vi "testFailIfEqual.vi"(8 "error in (no error)":errorcluster, 11 "MyFirstTest.lvclass in":refnum<class "MyFirstTest.lvclass">) -> (0 "error out":errorcluster, 3 "MyFirstTest.lvclass out":refnum<class "MyFirstTest.lvclass">)   [LabVIEW 2013, in "MyFirstTest.lvclass"]
doc: "This VI is a demo test -- it ensures that \"dog\" != \"cat\""
uses:
  MyFirstTest.lvclass
panel:
  # "Copyright © 2007 James Kring, Inc. All rights reserved.\n\nAuthor: Jim Kring [jim.kring@jameskring.com]\n\nThis library is provided \"AS IS\" ,WITHOUT WARRANTIES OR \nCONDITIONS OF ANY KIND, either express or implied.\n\nJames Kring, Inc. -- http://www.jameskring.com"
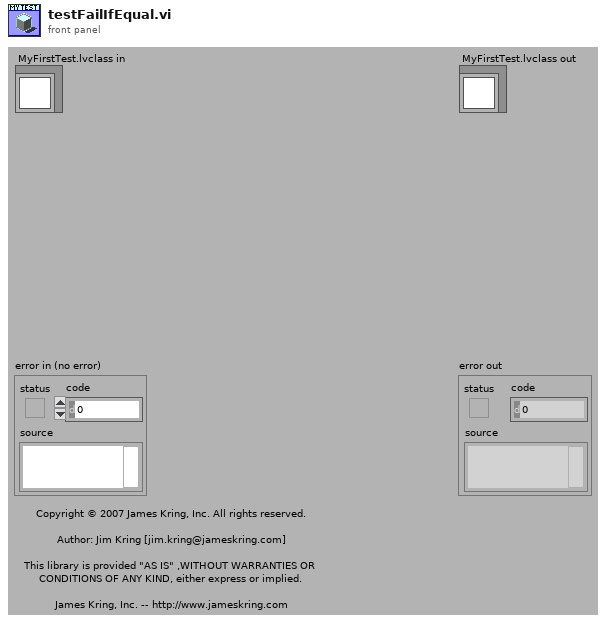
[diagram p1: front panel]
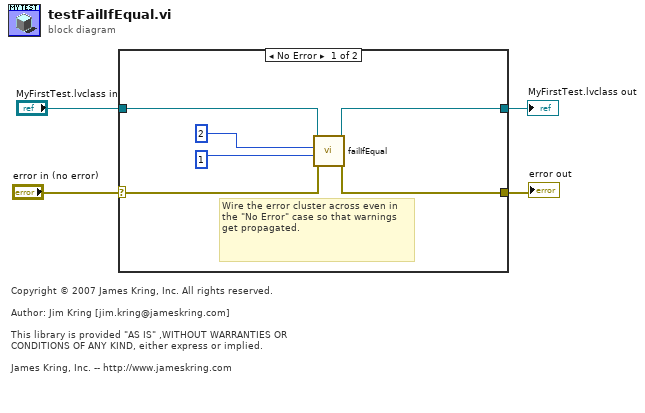
[diagram p0: block diagram]
diagram:
  # "Copyright © 2007 James Kring, Inc. All rights reserved.\n\nAuthor: Jim Kring [jim.kring@jameskring.com]\n\nThis library is provided \"AS IS\" ,WITHOUT WARRANTIES OR \nCONDITIONS OF ANY KIND, either express or implied.\n\nJames Kring, Inc. -- http://www.jameskring.com"
  n1 = case shown="No Error" "error in (no error)" {
    selector: "error in (no error)" -> [w8 w12]
    tunnel: [w7 w12] -> w3
    tunnel: [w9 w11] -> w1
    tunnel: "MyFirstTest.lvclass in" -> [w10 w11]
    frame No Error {
      # "Wire the error cluster across even in the \"No Error\" case so that warnings get propagated."
      n2 = call-dynamic "failIfEqual.vi"("error in (no error)"=w8, "y"=1, "x"=2, "TestCase in"=w10) -> ("error out"=w7:errorcluster, "TestCase out"=w9:refnum<class "MyFirstTest.lvclass">)  [unwired: 6 in]
    }
    frame Error {
    }
  }
  "error out" <- w3
  "MyFirstTest.lvclass out" <- w1
